vi "CANOpen_Enter SDO Information.vi"(8 "error in (no error)":errorcluster, 10 "SDO Parameters":T4[](array[typedef]) {"Sub-Index (0)" format="%.0x"; "Object Index" format="%.0x"; "Block Data" format="%.0x"}, 11 "Node Ptr":u64 format="%.0x") -> (0 "error out":errorcluster, 1 "Cancelled?":bool, 2 "SDO Parameters":T4[](array[typedef]) {"Sub-Index (0)" format="%.0x"; "Object Index" format="%.0x"; "Block Data" format="%.0x"}, 3 "Item Ref out":T5 format="%.0x")   [LabVIEW 2021, in "CANOpen Addon System Explorer.lvlib"]
uses:
  CANOpen Addon System Explorer.lvlib
  <vilib>/NI VeriStand/Custom Device API/Custom Device Item Ref.ctl
  Shared/CANOpen_SDO Settings.ctl
  Export.ctl
  CANOpen_SDO data format.ctl
  Import.ctl
  <vilib>/NI VeriStand/Custom Device API/Custom Device API.lvlib
  Shared/CANOpen Addon Shared.lvlib
panel:
  in  "Import SDO":T1
  in  "Cancel Button":bool
  in  "OK Button":bool
  in  "Import":T1
  in  "CSV data format":T2
  in  "Export":T3
  # "LSB"
  # "MSB"
  # "LSB"
  # "MSB"
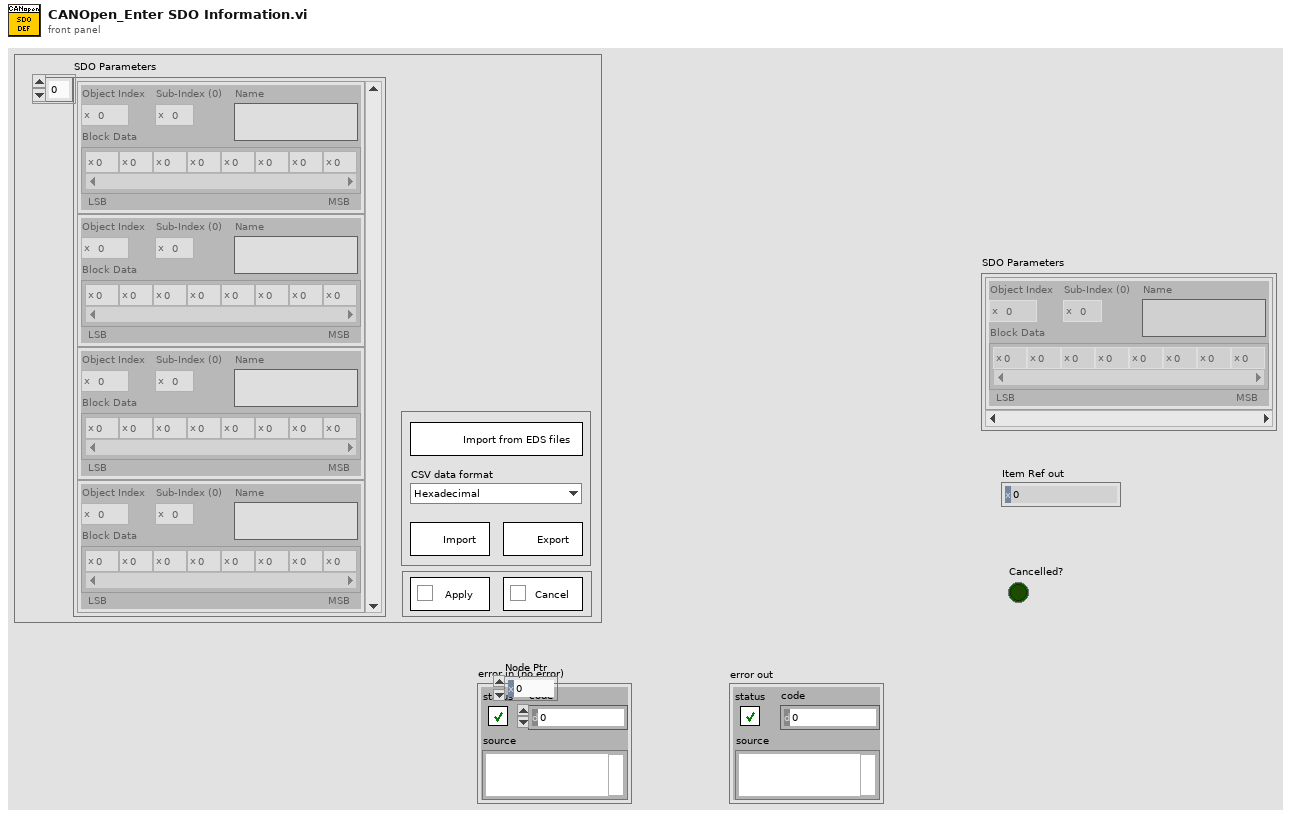
[diagram p1: front panel]
types:
  T1 = typedef "CANOpen Addon System Explorer.lvlib/Import.ctl" = bool
  T2 = typedef "CANOpen Addon System Explorer.lvlib/CANOpen_SDO data format.ctl" = enum16{"Hexadecimal", "Decimal"}
  T3 = typedef "CANOpen Addon System Explorer.lvlib/Export.ctl" = bool
  T4 = typedef "CANOpen Addon Shared.lvlib/CANOpen_SDO Settings.ctl" = cluster{"Object Index":u16, "Sub-Index (0)":u8, "Block Data":u8[], "Name":string}
  T5 = typedef "Custom Device API.lvlib/Custom Device Item Ref.ctl" = u64
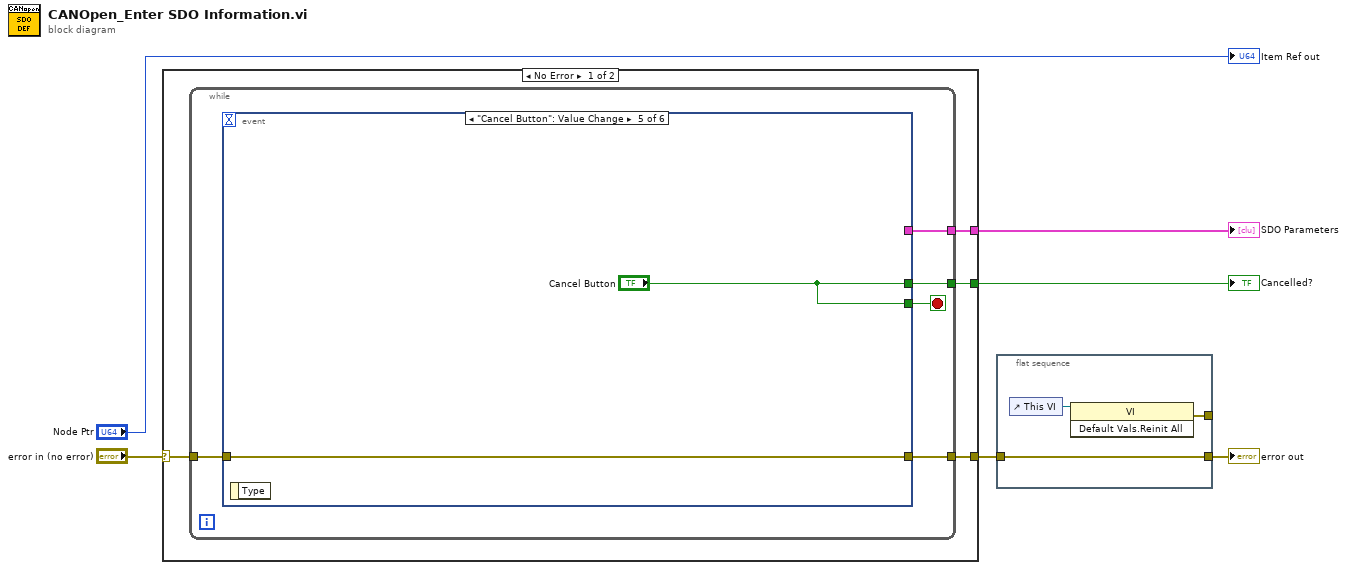
[diagram p0: block diagram]
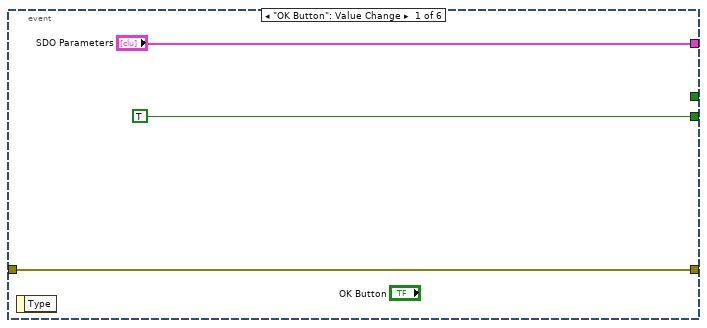
[diagram p2: hidden frame]
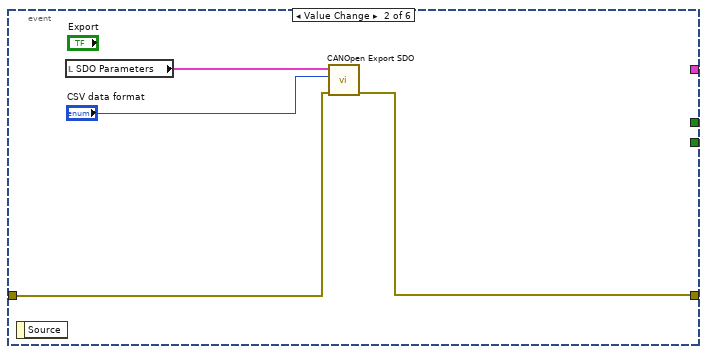
[diagram p3: hidden frame]
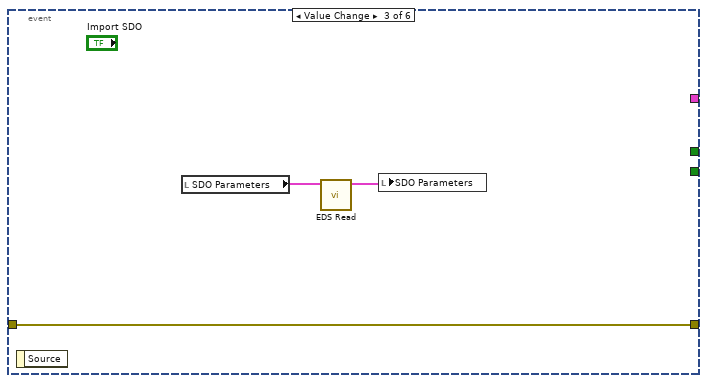
[diagram p4: hidden frame]
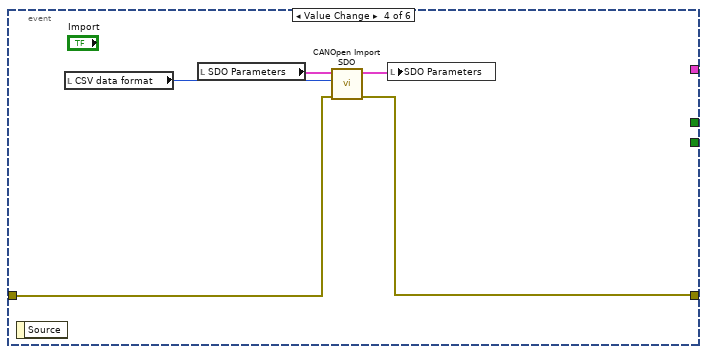
[diagram p5: hidden frame]
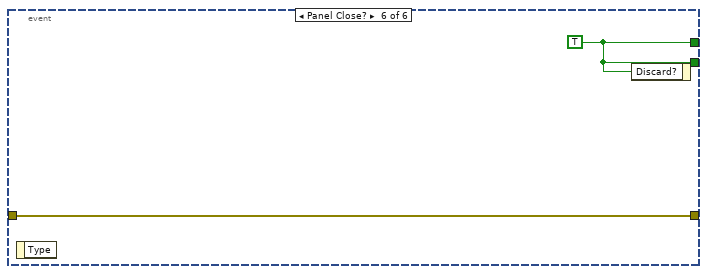
[diagram p6: hidden frame]
diagram:
  n1 = case shown="No Error" "error in (no error)" {
    selector: "error in (no error)" -> [w8 w35]
    tunnel: [w10 w35] -> w3
    tunnel: [w9 _] -> w6
    tunnel: [w7 _] -> w5
    frame No Error {
      n2 = while {
        tunnel: [w15] -> w10
        tunnel: w8 -> [w14]
        tunnel: [w12] -> w9
        tunnel: [w11] -> w7
        stop <- w13 stop-if-true
        n3 = event shown="[4] \"Cancel Button\": Value Change" {
          selector: _ -> [_ _ _ _ _ _]
          dyn-events: _ -> [_ _ _ _ _ _]
          timeout: _ -> [_ _ _ _ _ _]
          tunnel: [w18 w19 w23 w29 w32 w34] -> w15
          tunnel: w14 -> [w18 w20 w23 w30 w32 w34]
          tunnel: [TRUE ("Cancel Button") _ _ _ "Cancel Button" w33] -> w13
          tunnel: [_ _ _ _ "Cancel Button" w33] -> w12
          tunnel: ["SDO Parameters" _ _ _ _ _] -> w11
          event "OK Button": Value Change {
            n4 = event-data() -> ()  [unwired: 1 in, 1 out]
          }
          event Value Change {
            n5 = event-data() -> ()  [unwired: 1 in, 1 out]
            n6 = local read "SDO Parameters"() -> (w22:T4[])
            n7 = call "CANOpen Export SDO.vi"("error in (no error)"=w20, "Display format"="CSV data format", "SDO Parameters"=w22) -> ("error out"=w19:errorcluster)  [unwired: 8 in]
          }
          event Value Change {
            n8 = event-data() -> ()  [unwired: 1 in, 1 out]
            n9 = local read "SDO Parameters"() -> (w25:T4[])
            n10 = call "EDS Read.vi"("SDO Parameters"=w25) -> ("SDO Parameters out"=w24:T4[])  [unwired: 10 in]
            n11 = local write "SDO Parameters"(w24) -> ()
          }
          event Value Change {
            n12 = event-data() -> ()  [unwired: 1 in, 1 out]
            n13 = local read "CSV data format"() -> (w28:T2)
            n14 = local read "SDO Parameters"() -> (w26:T4[])
            n15 = call "CANOpen Import SDO.vi"("error in (no error)"=w30, "Display format"=w28, "SDO Parameters in"=w26) -> ("error out"=w29:errorcluster, "SDO Parameters"=w27:T4[])  [unwired: 7 in]
            n16 = local write "SDO Parameters"(w27) -> ()
          }
          event "Cancel Button": Value Change {
            n17 = event-data() -> ()  [unwired: 1 in, 1 out]
          }
          event Panel Close? {
            w33 = TRUE ("Cancel Button")
            n18 = event-data() -> ()  [unwired: 1 in, 1 out]
            n19 = event-data("Discard?"=w33) -> ()  [unwired: 1 in, 1 out]
          }
        }
      }
    }
    frame Error {
    }
  }
  "Cancelled?" <- w6
  "SDO Parameters" <- w5
  n20 = flat-sequence {
    tunnel: [w38] -> w4
    tunnel: w3 -> [w38]
    tunnel: [w36] -> _
    frame #0 {
      n21 = control-ref of="This VI"() -> (w37:refnum<vi>)
      n22 = invoke class="VI" method="Default Vals.Reinit All"(reference=w37) -> (error out=w36:errorcluster)  [unwired: 2 in, 2 out]
    }
  }
  "error out" <- w4
  "Item Ref out" <- "Node Ptr"
